vi "IP Generator.vi"(3 "String":string) -> (1 "Array":string[](array[string]))   [LabVIEW 2024]
uses:
  <vilib>/Analysis/1siggen.llb/Ramp Pattern by Samples.vi
  <vilib>/Analysis/NI_AALBase.lvlib
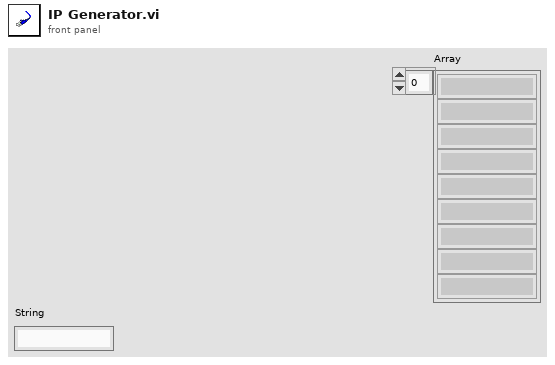
[diagram p1: front panel]
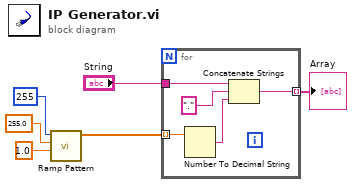
[diagram p0: block diagram]
diagram:
  n1 = call-poly <vilib>:"Ramp Pattern.vi"("start"=1.0, "end"=255.0, "samples"=255) -> ("Ramp Pattern"=w3:dbl[])  [unwired: 7 in, 1 out]
  n2 = for {
    tunnel: w3 -> [w11] mode=indexing
    tunnel: "String" -> [w9]
    tunnel: [w10] -> w1 mode=indexing
    n3 = Number To Decimal String(number=w11) -> (decimal integer string=w7:string)  [unwired: 1 in]
    n4 = Concatenate Strings(w9, "." ("string"), w7) -> (w10:string)
  }
  "Array" <- w1
